vi "Package Typed Message.vi"(8 "error in (no error)":errorcluster, 11 "Group in":refnum<class "Group DBL.lvclass">) -> (0 "error out":errorcluster, 2 "Data Msg":refnum<class "Message.lvclass">, 3 "Group out":refnum<class "Group DBL.lvclass">)   [LabVIEW 2020, in "Vecto.lvlib" / "Group DBL.lvclass"]
uses:
  Group DBL.lvclass
  C:/dev/lv20CE/relink/lv-vecto/Vecto/Group/Group.lvclass
  lv-protoc/LV-Proto/Message/Message.lvclass
  Group/Group.lvclass/Group.ctl
  Group DBL.lvclass/Group DBL.ctl
  Group Config/Group Config.lvclass/Group Config.ctl
  proto/GroupData/Class/Msg.lvclass/Msg.ctl
  Double to Relative ns.vi
  proto/GroupData/Class/Msg.lvclass
  C:/dev/lv20CE/relink/lv-protoc/LV-Proto/Message/Message.lvclass
  Group Config/Group Config.lvclass
  Group/Group.lvclass
  Vecto.lvlib
  C:/dev/lv20CE/relink/lv-vecto/Vecto/Group DBL/Group DBL.lvclass
  lv-volatus/messages/DoubleData/Data.ctl
  lv-volatus/messages/DoubleData/DoubleData.lvlib
  lv-volatus/messages/DoubleData/Class/Msg.lvclass
  C:/dev/lv20CE/relink/lv-volatus/messages/DoubleData/Class/Msg.lvclass
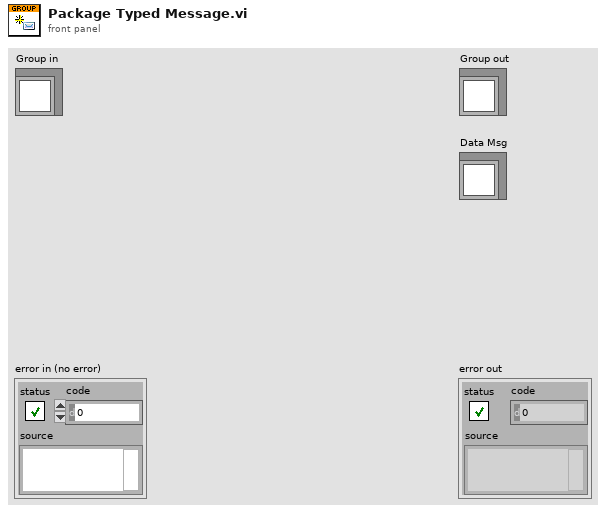
[diagram p1: front panel]
types:
  T1 = typedef "DoubleData.lvlib/Data.ctl" = cluster{"group_name":string, "data_timestamp":i64, "scaled_data":dbl[], "raw_data":dbl[], "names_crc":u32}
  T2 = typedef "Vecto.lvlib/Group.lvclass/Ref.ctl" = cluster{"Scaled":dbl[], "Timestamp":dbl[], "Raw":dbl[]}
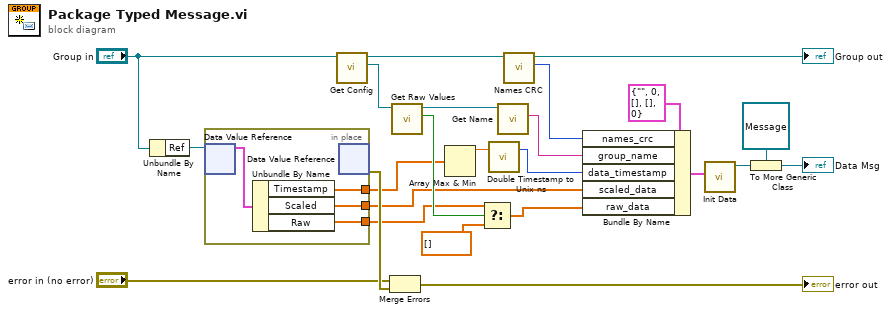
[diagram p0: block diagram]
diagram:
  n1 = Unbundle By Name("Group in") -> ("Ref"=w21:refnum<data-value>)
  n2 = in-place {
    in-place-border: [w27] -> w8
    in-place-border: [w26] -> w9
    in-place-border: [w25] -> w7
    n3 = in-place-dvr #1(w21) -> (w28:T2)  [unwired: 1 out]
    n4 = Unbundle By Name(w28) -> ("Timestamp"=w26:dbl[], "Scaled"=w27:dbl[], "Raw"=w25:dbl[])
    n5 = in-place-dvr #1() -> (w24:errorcluster)  [unwired: 1 in, 1 out]
  }
  n6 = call "Get Config.vi"("Group in"="Group in") -> ("Config"=w5:refnum<class "Group Config.lvclass">, "Group out"=w6:refnum<class "Group DBL.lvclass">)  [unwired: 8 in, 1 out]
  n7 = Merge Errors("error in (no error)", w24) -> (→"error out":errorcluster)
  n8 = call "Get Raw Values.vi"("Group Config in"=w5) -> ("Raw Values"=w14:bool, "Group Config out"=w13:refnum<class "Group Config.lvclass">)  [unwired: 8 in, 1 out]
  n9 = Array Max & Min(array=w9) -> (max value=w19:dbl)  [unwired: 3 out]
  n10 = Select(t=w7, s=w14, f=dbl[] []) -> (s? t:f=w15:dbl[])
  n11 = call "Double Timestamp to Unix ns.vi"("Timestamp"=w19) -> ("unix ns"=w18:i64)  [unwired: 2 in]
  n12 = call "Get Name.vi"("Group Config in"=w13) -> ("Name"=w12:string)  [unwired: 8 in, 2 out]
  n13 = call "Names CRC.vi"("Group in"=w6) -> ("Names CRC"=w1:u32, "Group out"=→"Group out":refnum<class "Group DBL.lvclass">)  [unwired: 9 in]
  n14 = Bundle By Name(cluster=T1 {"group_name"="", "data_timestamp"=0, "scaled_data"=[], "raw_data"=[], "names_crc"=0} ("GroupData"), "names_crc"=w1, "group_name"=w12, "data_timestamp"=w18, "scaled_data"=w8, "raw_data"=w15) -> (w11:T1)
  n15 = call "Init Data.vi"("Data"=w11) -> ("Msg out"=w10:refnum<class "Msg.lvclass">)  [unwired: 10 in]
  n16 = To More Generic Class(target class=refnum<class "Message.lvclass"> refnum ("LV-Proto.lvlib:Message.lvclass"), reference=w10) -> (generic class reference=→"Data Msg":refnum<class "Message.lvclass">)
